vi "OC2 Read Output.vi"(3 "error in (no error)":errorcluster, 4 "output report in":T1 {"Output freq." format="%.1f"; "Output" items=["Negative", "Positive"]}, 5 "enable":bool, 6 "VISA resource name":refnum<visa-resource-name>) -> (0 "error out":errorcluster, 1 "output report out":T1 {"Output freq." format="%.1f"; "Output" items=["Negative", "Positive"]}, 2 "dup VISA resource name":refnum<visa-resource-name>)   [LabVIEW 2009]
doc: "TCM Read Output.vi\n\nVI that Reads the output information, accepts a cluster that contains the following variables:\nOutput - negative or positive output\nOutput min % - minimum output percentage allowed\nOutput max % - maximum output percentage allowed\nOutput freq - frequency of the PWM output signal\n\nCOPYRIGHT ELECTRON DYNAMICS LTD"
panel:
  in  "Command":string
  out "Rx string":string
  # "Read output"
  # "V1.02"
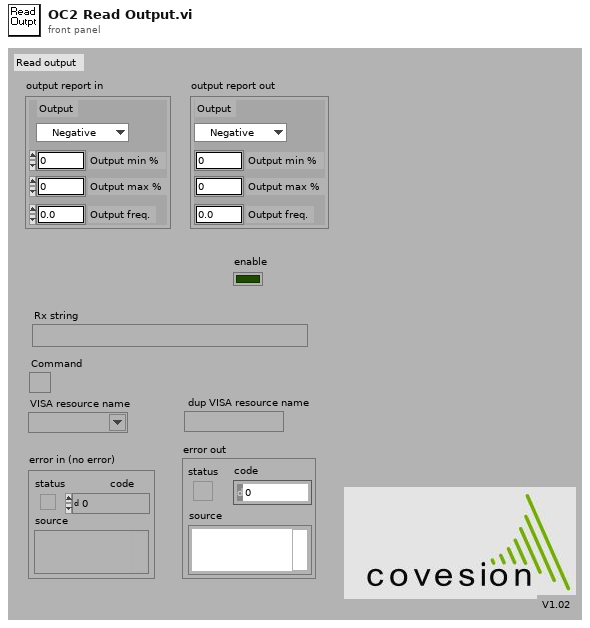
[diagram p1: front panel]
types:
  T1 = cluster{"Output":u16, "Output min %":dbl, "Output max %":dbl, "Output freq.":dbl}
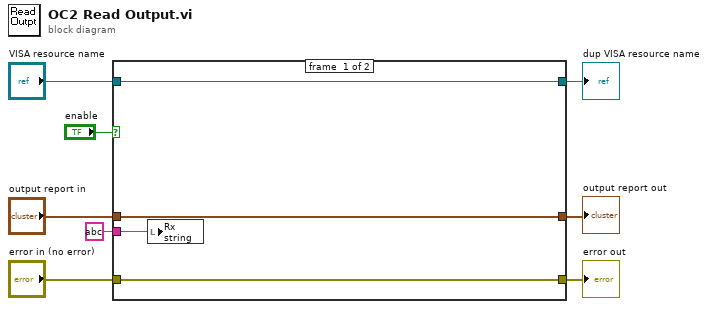
[diagram p0: block diagram]
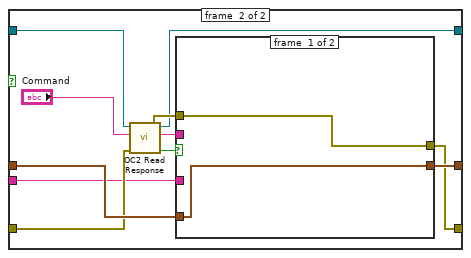
[diagram p2: hidden frame]
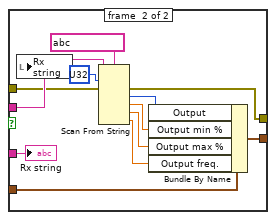
[diagram p3: hidden frame]
diagram:
  n1 = case shown="True" "enable" {
    tunnel: "output report in" -> [w11 w21]
    tunnel: "VISA resource name" -> [w12 w20]
    tunnel: "error in (no error)" -> [w10 w19]
    tunnel: [w11 w16] -> w5
    tunnel: [w10 w15] -> w4
    tunnel: [w12 w14] -> w3
    tunnel: string ? -> [w9 w13]
    frame #0 {
      n2 = local write "Rx string"(w9) -> ()
    }
    frame #1 {
      n3 = call "OC2 Read Response.vi"("error in (no error)"=w19, "Command"="Command", "VISA resource name"=w20) -> ("RX packet ok"=w18:bool, "error out"=w17:errorcluster, "output string"=w23:string, "dup VISA resource name"=w14:refnum<visa-resource-name>)  [unwired: 1 in]
      n4 = case shown="True" w18 {
        tunnel: w23 -> [_ w35]
        tunnel: w21 -> [w25 w34]
        tunnel: w17 -> [w24 w29]
        tunnel: [w25 w28] -> w16
        tunnel: [w24 w27] -> w15
        tunnel: w13 -> [_ w26]
        frame #0 {
        }
        frame #1 {
          n5 = local write "Rx string"(w35) -> ()
          n6 = Scan From String(format string=string ?, input string=w35, initial scan location=u32 ?, error in=w29) -> (error out=w27:errorcluster, output 1=w33:i32, output 2=w32:dbl, output 3=w31:dbl, output 4=w30:dbl)  [unwired: 4 in, 2 out]
          n7 = Bundle By Name(cluster=w34, "Output"=w33, "Output min %"=w32, "Output max %"=w31, "Output freq."=w30) -> (w28:T1)
          "Rx string" <- w26
        }
      }
    }
  }
  "dup VISA resource name" <- w3
  "error out" <- w4
  "output report out" <- w5
